vi "MPU_Stick_Write_Configuration_Parameter.vi"(0 "ADCP in":refnum<class "ADCP.lvclass">, 5 "Parameter Name":string, 7 "Parameter Value":string, 9 "Write Enable Parameter Name":string, 11 "error out":errorcluster) -> (4 "ADCP out":refnum<class "ADCP.lvclass">, 6 "Result":bool, 15 "error out":errorcluster)   [LabVIEW 2017]
uses:
  Classes/ADCP.lvclass
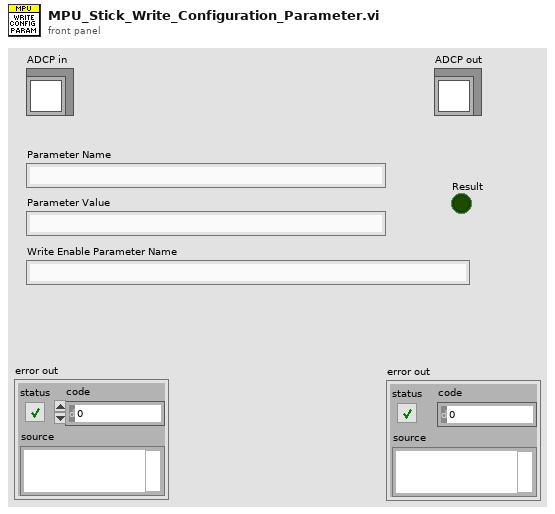
[diagram p1: front panel]
types:
  T1 = cluster{"Parameter name":string, "Node name":string, "Node ID":u8, "Frame name":string, "Frame ID":u8, "Start bit":u32, "Bit length":u32, "Factor":dbl, "Offset":dbl, "Minimum":dbl, "Maximum":dbl, "Value":string, "Comments":string, "Data_Type":enum16{"BOOL", "UNSIGNED", "SIGNED", "FLOAT32", "ENUM"}, "Enum List":string[]}[]
  T2 = cluster{"Parameter name":string, "Node name":string, "Node ID":u8, "Frame name":string, "Frame ID":u8, "Start bit":u32, "Bit length":u32, "Factor":dbl, "Offset":dbl, "Minimum":dbl, "Maximum":dbl, "Value":string, "Comments":string, "Data_Type":enum16{"BOOL", "UNSIGNED", "SIGNED", "FLOAT32", "ENUM"}, "Enum List":string[]}
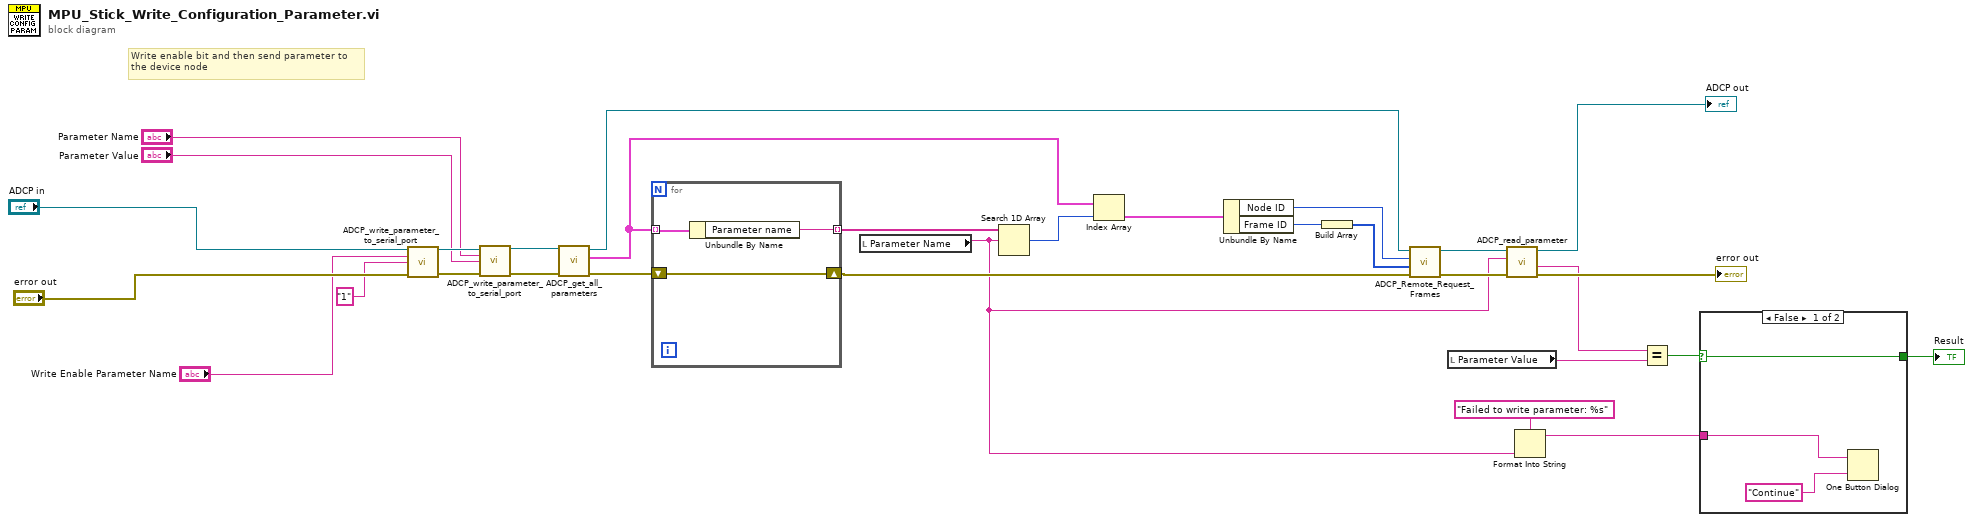
[diagram p0: block diagram]
diagram:
  # "Write enable bit and then send parameter to\nthe device node"
  n1 = call "ADCP_write_parameter_to_serial_port.vi"("ADCP In"="ADCP in", "Parameter name"="Write Enable Parameter Name", "Parameter value"="1" ("Parameter Value"), "error in (no error)"="error out") -> ("ADCP out"=w8:refnum<class "ADCP.lvclass">, "error out"=w7:errorcluster)  [unwired: 8 in, 2 out]
  n2 = call "ADCP_write_parameter_to_serial_port.vi"("ADCP In"=w8, "Parameter name"="Parameter Name", "Parameter value"="Parameter Value", "error in (no error)"=w7) -> ("ADCP out"=w5:refnum<class "ADCP.lvclass">, "error out"=w4:errorcluster)  [unwired: 8 in, 2 out]
  n3 = call "ADCP_get_all_parameters.vi"("error in (no error)"=w4, "ADCP In"=w5) -> ("error out"=w31:errorcluster, "Parameters"=w29:T1, "ADCP Out"=w22:refnum<class "ADCP.lvclass">)  [unwired: 6 in, 1 out]
  n4 = for {
    shift-right: [w32] -> w23
    shift-left: w31 -> [w32]
    tunnel: w29 -> [w34] mode=indexing
    tunnel: [w33] -> w30 mode=indexing
    n5 = Unbundle By Name(w34) -> ("Parameter name"=w33:string)
  }
  n6 = local read "Parameter Name"() -> (w12:string)
  n7 = Search 1D Array(1D array=w30, element=w12) -> (index of element=w28:i32)  [unwired: 1 in]
  n8 = Index Array(array=w29, index=w28) -> (element=w27:T2)
  n9 = Unbundle By Name(w27) -> ("Node ID"=w24:u8, "Frame ID"=w26:u8)
  n10 = Build Array(w26) -> (w25:u8[])
  n11 = call "ADCP_Remote_Request_Frames.vi"("error in (no error)"=w23, "Request Frame IDs"=w25, "Node ID"=w24, "ADCP In"=w22) -> ("error out"=w20:errorcluster, "ADCP Out"=w21:refnum<class "ADCP.lvclass">)  [unwired: 4 in, 2 out]
  n12 = local read "Parameter Value"() -> (w16:string)
  n13 = call "ADCP_read_parameter.vi"("error in (no error)"=w20, "Parameter Name"=w12, "ADCP In"=w21) -> ("error out"=→"error out":errorcluster, "Parameter Value"=w17:string, "ADCP out"=→"ADCP out":refnum<class "ADCP.lvclass">)  [unwired: 5 in, 1 out]
  n14 = Format Into String(format string="Failed to write parameter: %s", w12) -> (resulting string=w11:string)  [unwired: 2 in, 1 out]
  n15 = Equal?(x=w17, y=w16) -> (x = y?=w15:bool)
  n16 = case shown="False" w15 {
    selector: w15 -> [w37 w38]
    tunnel: [w37 w38] -> w14
    tunnel: w11 -> [w35 _]
    frame False {
      n17 = One Button Dialog(message=w35, button name ("OK")="Continue") -> ()  [unwired: 1 out]
    }
    frame True {
    }
  }
  "Result" <- w14
